vi "setFPGAReference.vi"(10 "FPGAReference":refnum<k20>, 11 "SoftwareControlledTrigger in":refnum<class "SoftwareControlledTrigger.lvclass">) -> (3 "SoftwareControlledTrigger out":refnum<class "SoftwareControlledTrigger.lvclass">)   [LabVIEW 2016, in "SoftwareControlledTrigger.lvclass"]
uses:
  SoftwareControlledTrigger.lvclass
  SoftwareControlledTrigger.lvclass/SoftwareControlledTrigger.ctl
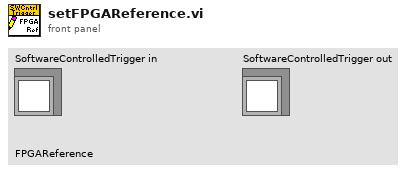
[diagram p1: front panel]
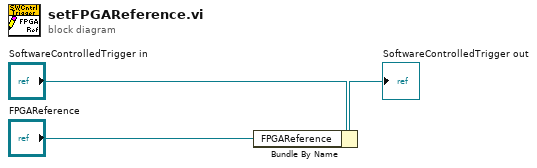
[diagram p0: block diagram]
diagram:
  n1 = Bundle By Name(cluster="SoftwareControlledTrigger in", "FPGAReference"="FPGAReference") -> (→"SoftwareControlledTrigger out":refnum<class "SoftwareControlledTrigger.lvclass">)
